vi "QTrkGenerateGaussian2DSpot.vi"(0 "Position":cluster{"X":sgl, "Y":sgl}, 1 "Width":i32=32, 2 "Height":i32=32, 5 "sigma":sgl=4.0, 7 "I0":sgl=2000.0, 9 "Ibg":sgl=5.0, 11 "Apply poisson noise?":bool) -> (4 "Image":sgl[][](array[numeric]))   [LabVIEW 2011]
uses:
  QTrkDLL.vi
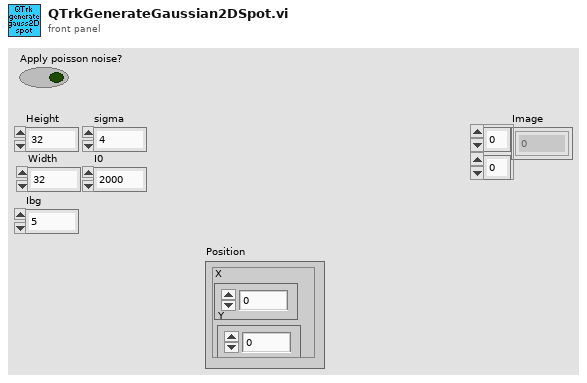
[diagram p1: front panel]
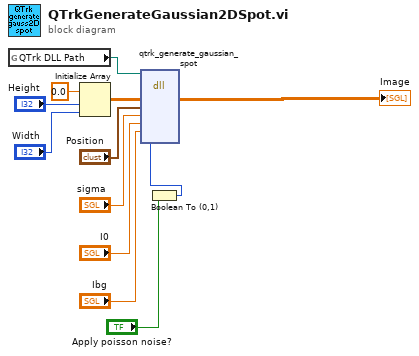
[diagram p0: block diagram]
diagram:
  n1 = global read "QTrkDLL.vi" "QTrk DLL Path"() -> (w3:path)
  n2 = Initialize Array(sgl 0.0 ("element"), "Height", "Width") -> (w8:sgl[][])
  n3 = Boolean To (0,1)(Boolean="Apply poisson noise?") -> (0, 1=w2:i16)
  n4 = dll-call lib="D:/jcnossen1/cudaqi-tracker/qtrk/lv/qtrk-labview.dll" fn="qtrk_generate_gaussian_spot"(path in=w3, "image"=w8, "position"="Position", "sigma"="sigma", "I0"="I0", "Ibg"="Ibg", "applyNoise"=w2) -> ("image"=→"Image":sgl[][])  [unwired: 8 in, 2 out]
